vi "Initialize txt file for NOK tests from previous DUT.vi"() -> (0 "error out":errorcluster)   [LabVIEW 2023, in "In a row NOK.lvlib"]
uses:
  In a row NOK.lvlib
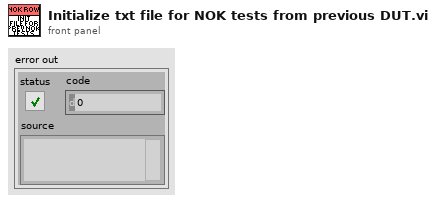
[diagram p1: front panel]
types:
  T1 = enum16{"open", "replace", "create", "open or create", "replace or create", "replace or create with confirmation"}
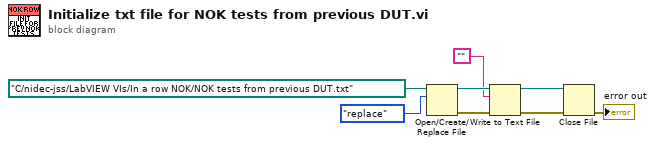
[diagram p0: block diagram]
diagram:
  n1 = Open/Create/Replace File(file path (use dialog)=path "C:/nidec-jss/LabVIEW VIs/In a row NOK/NOK tests from previous DUT.txt", operation (0:open)=T1."replace") -> (refnum out=w7:refnum<file>, error out=w6:errorcluster)  [unwired: 4 in, 1 out]
  n2 = Write to Text File(file (use dialog)=w7, text="", error in=w6) -> (refnum out=w5:refnum<file>, error out=w4:errorcluster)  [unwired: 1 in, 1 out]
  n3 = Close File(refnum=w5, error in=w4) -> (error out=→"error out":errorcluster)  [unwired: 1 out]
